vi "Output_single_waveform.vi"() -> ()   [LabVIEW 2019]
uses:
  Create_waveform/build_waveform.lvclass
  Write_to_file/Write_to_file.lvclass
  Plot_waveform/Plot_waveform.lvclass
panel:
  in  "Amplitude":dbl=127.0 format="%#_13g"
  out "Waveform":waveform(dbl)(graph)={"t0"=timestamp(0 s since 1904-01-01), "dt"=8.333333333333334e-10, "Y"=array[8192 elements]}
  in  "start path":path=path "C:/GitHub/PulseEcho/PulsedFieldEcho/Create_Pulse"
  in  "standard deviation":dbl=0.1
  in  "NWaves":i32=75
  in  "Frequency":dbl=217000000.0
  in  "clock rate":dbl=1200000000.0 format="%#_6p"
  # "Select Path"
  # "Pulse Parameters"
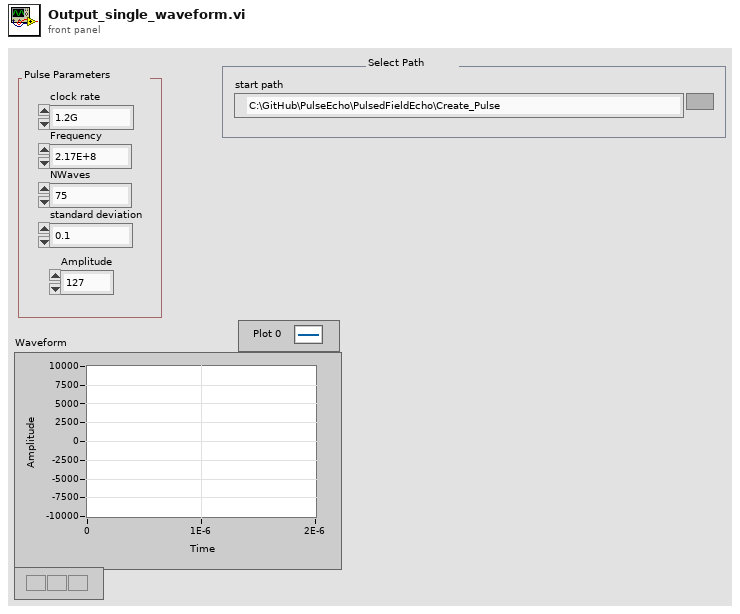
[diagram p1: front panel]
types:
  T1 = enum16{"open", "replace", "create", "open or create", "replace or create", "replace or create with confirmation"}
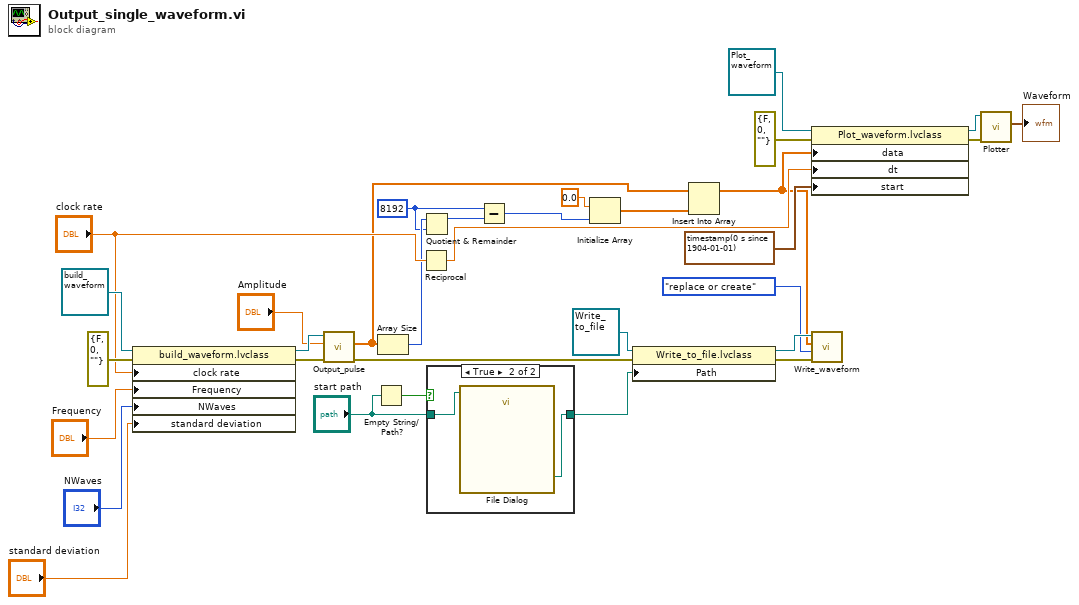
[diagram p0: block diagram]
diagram:
  w10 = 8192
  n1 = property class="build_waveform.lvclass"(reference=refnum<class "build_waveform.lvclass"> refnum ("build_waveform.lvclass"), error in=errorcluster {"status"=FALSE, "code"=0, "source"=""} ("error in (no error)"), "clock rate"="clock rate", "Frequency"="Frequency", "NWaves"="NWaves", "standard deviation"="standard deviation") -> (reference out=w27:refnum<class "build_waveform.lvclass">, error out=w26:errorcluster)
  n2 = call-dynamic "Output_pulse.vi"("error in (no error)"=w26, "Amplitude"="Amplitude", "build_waveform in"=w27) -> ("error out"=w13:errorcluster, "Array"=w5:dbl[])  [unwired: 6 in, 1 out]
  n3 = Empty String/Path?(string/path="start path") -> (empty?=w1:bool)
  n4 = Array Size(array=w5) -> (size(s)=w11:i32)
  n5 = Reciprocal(x="clock rate") -> (1/x=w22:dbl)
  n6 = Quotient & Remainder(x=w11, y=w10) -> (x-y*floor(x/y)=w9:i32)  [unwired: 1 out]
  n7 = case shown="True" w1 {
    tunnel: [w33 w35] -> w25
    tunnel: "start path" -> [w33 w34]
    frame False {
    }
    frame True {
      n8 = call "File Dialog"("start path"=w34) -> ("selected path"=w35:path)  [unwired: 11 in, 3 out]
    }
  }
  n9 = Subtract(x=w10, y=w9) -> (x-y=w6:i32)
  n10 = Initialize Array(0.0 ("element"), w6) -> (w7:dbl[])
  n11 = property class="Write_to_file.lvclass"(reference=refnum<class "Write_to_file.lvclass"> refnum ("Write_to_file.lvclass"), error in=w13, "Path"=w25) -> (reference out=w14:refnum<class "Write_to_file.lvclass">, error out=w16:errorcluster)
  n12 = Insert Into Array(array=w5, new element=w7) -> (w4:dbl[])  [unwired: 1 in]
  n13 = property class="Plot_waveform.lvclass"(reference=refnum<class "Plot_waveform.lvclass"> refnum ("Plot_waveform.lvclass"), error in=errorcluster {"status"=FALSE, "code"=0, "source"=""} ("error in (no error)"), "data"=w4, "dt"=w22, "start"=timestamp(0 s since 1904-01-01)) -> (reference out=w20:refnum<class "Plot_waveform.lvclass">, error out=w19:errorcluster)
  n14 = call-dynamic "Write_waveform.vi"("error in (no error)"=w16, "operation (0:open)"=T1."replace or create", "Array"=w4, "Write_to_file in"=w14) -> ()  [unwired: 6 in, 2 out]
  n15 = call-dynamic "Plotter.vi"("error in (no error)"=w19, "Plot_waveform in"=w20) -> ("output waveform"=→"Waveform":waveform(dbl))  [unwired: 7 in, 2 out]
